vi "test_Create FPGA Addon_Error.vi"(8 "error in (no error)":errorcluster, 11 "TestCase in":refnum<class "FPGA Addon Scripting API Unit Tests.lvclass">) -> (0 "error out":errorcluster, 3 "TestCase out":refnum<class "FPGA Addon Scripting API Unit Tests.lvclass">)   [LabVIEW 2018, in "FPGA Addon Scripting API Unit Tests.lvclass"]
uses:
  FPGA Addon Scripting API Unit Tests.lvclass
  <vilib>/addons/_JKI Toolkits/VI Tester/TestCase.llb/TestCase.lvclass
  FPGA Addon Test Class/FPGA Addon Test Class.lvclass
  APIs/Scripting API/Scripting API.lvlib
  C:/Program Files (x86)/National Instruments/LabVIEW 2018/vi.lib/addons/_JKI Toolkits/VI Tester/TestCase.llb/TestCase.lvclass
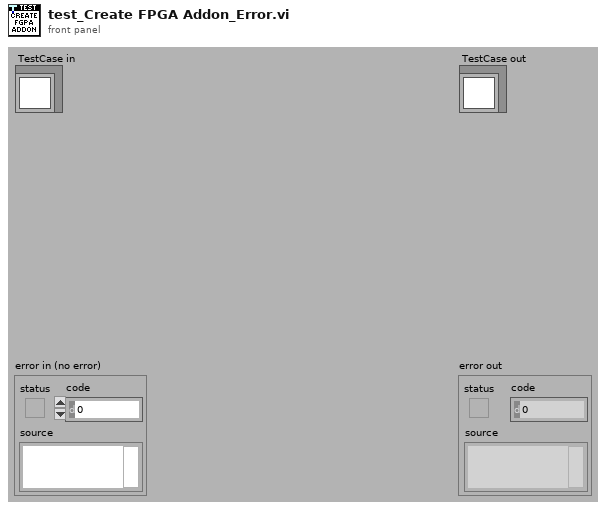
[diagram p1: front panel]
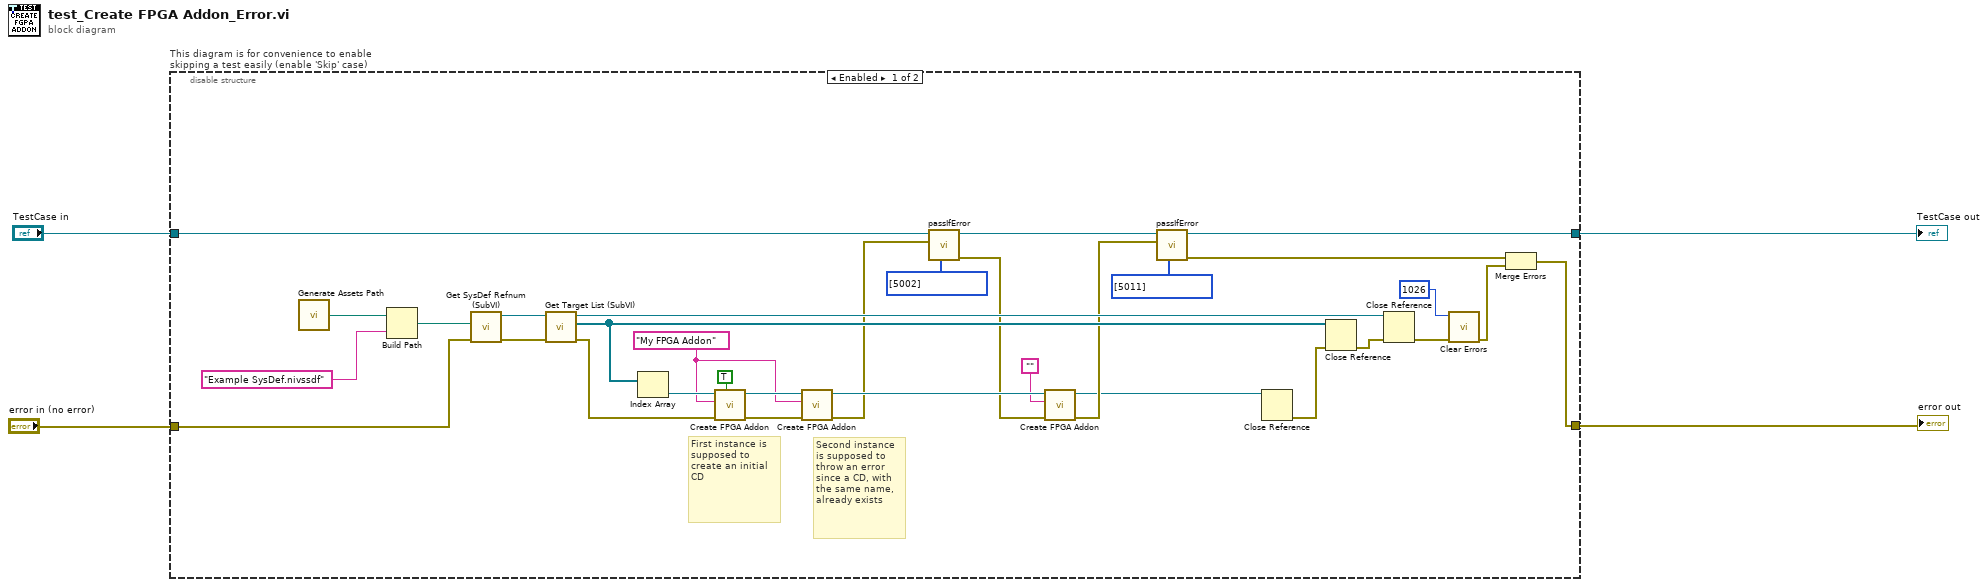
[diagram p0: block diagram]
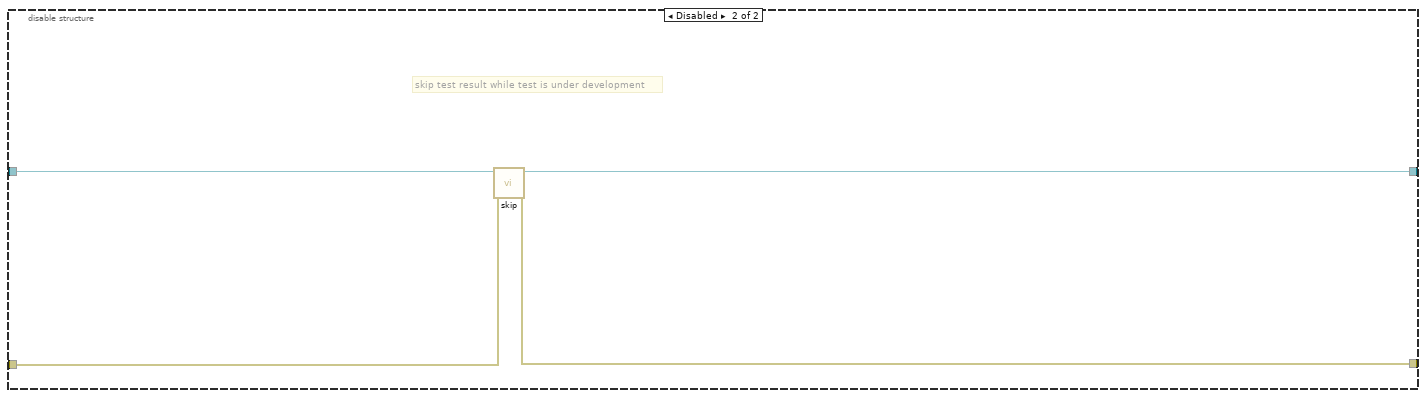
[diagram p2: hidden frame]
diagram:
  n1 = disable-structure "This diagram is for convenience to enable skipping a test easily (enable 'Skip' case)" shown="Enabled" {
    disable-tunnel: "TestCase in" -> [w20 w40]
    disable-tunnel: [w11 w38] -> w1
    disable-tunnel: [w8 w39] -> w3
    disable-tunnel: "error in (no error)" -> [w31 w37]
    frame Enabled {
      w22 = "My FPGA Addon" ("FPGA addon name")
      # "Second instance is supposed to throw an error since a CD, with the same name, already exists"
      # "First instance is supposed to create an initial CD"
      n2 = call "Generate Assets Path.vi"() -> ("Assets path"=w36:path)
      n3 = Build Path(base path=w36, name or relative path="Example SysDef.nivssdf") -> (appended path=w34:path)
      n4 = call "Get SysDef Refnum (SubVI).vi"("error in (no error)"=w31, "System Definition path"=w34) -> ("error out"=w30:errorcluster, "SysDef Refnum out"=w33:refnum<k24>)  [unwired: 8 in]
      n5 = call "Get Target List (SubVI).vi"("error in (no error)"=w30, "SysDef Refnum in"=w33) -> ("error out"=w29:errorcluster, "Target List Refnums"=w28:refnum<k24>[], "SysDef Refnum out"=w27:refnum<k24>)  [unwired: 7 in]
      n6 = Index Array(array=w28) -> (element=w32:refnum<k24>)  [unwired: 1 in]
      n7 = call "Create FPGA Addon.vi"("group scalars"=TRUE, "error in"=w29, "FPGA addon name"=w22, "target in"=w32) -> ("error out"=w24:errorcluster, "target out"=w23:refnum<k24>)  [unwired: 5 in, 1 out]
      n8 = call "Create FPGA Addon.vi"("error in"=w24, "FPGA addon name"=w22, "target in"=w23) -> ("error out"=w15:errorcluster, "target out"=w17:refnum<k24>)  [unwired: 6 in, 1 out]
      n9 = call-dynamic "passIfError.vi"("passing error codes (default = any error code)"=i32[] [5002], "error"=w15, "TestCase in"=w20) -> ("error out"=w14:errorcluster, "TestCase out"=w18:refnum<class "FPGA Addon Scripting API Unit Tests.lvclass">)  [unwired: 7 in]
      n10 = call "Create FPGA Addon.vi"("error in"=w14, "FPGA addon name"="", "target in"=w17) -> ("error out"=w13:errorcluster, "target out"=w10:refnum<k24>)  [unwired: 6 in, 1 out]
      n11 = call-dynamic "passIfError.vi"("passing error codes (default = any error code)"=i32[] [5011], "error"=w13, "TestCase in"=w18) -> ("error out"=w9:errorcluster, "TestCase out"=w11:refnum<class "FPGA Addon Scripting API Unit Tests.lvclass">)  [unwired: 7 in]
      n12 = Close Reference(reference=w10) -> (error out=w21:errorcluster)  [unwired: 1 in]
      n13 = Close Reference(reference=w28, error in (no error)=w21) -> (error out=w26:errorcluster)
      n14 = Close Reference(reference=w27, error in (no error)=w26) -> (error out=w7:errorcluster)
      n15 = call <vilib>:"Clear Errors.vi"("error in (no error)"=w7, "specific error code to clear (0: all)"=1026) -> ("error out"=w6:errorcluster)  [unwired: 4 in, 1 out]
      n16 = Merge Errors(w9, w6) -> (w8:errorcluster)
    }
    frame Disabled {
      # "skip test result while test is under development"
      n17 = call <vilib>:"skip.vi"("error in (no error)"=w37, "TestCase in"=w40) -> ("error out"=w39:errorcluster, "TestCase out"=w38:refnum<class "FPGA Addon Scripting API Unit Tests.lvclass">)  [unwired: 8 in]
    }
  }
  "error out" <- w3
  "TestCase out" <- w1
